vi "CalcArmCurlSpeed.vi"(9 "Curl Speed":dbl, 10 "Arm Down":bool, 11 "Arm Up":bool) -> (2 "Arm Speed":dbl, 3 "Shoulder Speed":dbl)   [LabVIEW 2018]
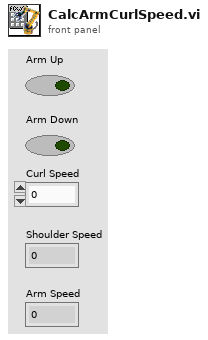
[diagram p1: front panel]
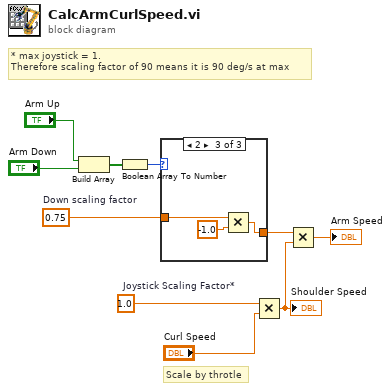
[diagram p0: block diagram]
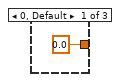
[diagram p2: hidden frame]
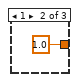
[diagram p3: hidden frame]
diagram:
  w1 = 0.75  # Down scaling factor
  w10 = 1.0  # Joystick Scaling Factor*
  # "Scale by throtle"
  # "* max joystick = 1.\nTherefore scaling factor of 90 means it is 90 deg/s at max"
  n1 = Build Array("Arm Up", "Arm Down") -> (w8:bool[])
  n2 = Boolean Array To Number(Boolean array=w8) -> (number=w5:u32)
  n3 = case shown="2" w5 {
    tunnel: [0.0 1.0 w14] -> w4
    tunnel: w1 -> [_ _ w13]
    frame 0, Default {
    }
    frame 1 {
    }
    frame 2 {
      n4 = Multiply(x=w13, y=-1.0) -> (x*y=w14:dbl)
    }
  }
  n5 = Multiply(x=w10, y="Curl Speed") -> (x*y=w2:dbl)
  "Shoulder Speed" <- w2
  n6 = Multiply(x=w4, y=w2) -> (x*y=→"Arm Speed":dbl)
